vi "Test single channel GPU FFT.vi"() -> ()   [LabVIEW 2018]
panel:
  in  "stop":bool
  out "Waveform Chart":dbl(graph)
  out "error out":errorcluster
  in  "error in (no error)":errorcluster
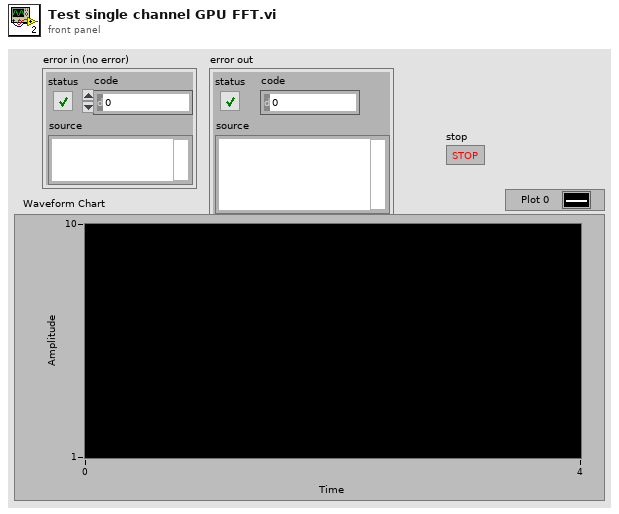
[diagram p1: front panel]
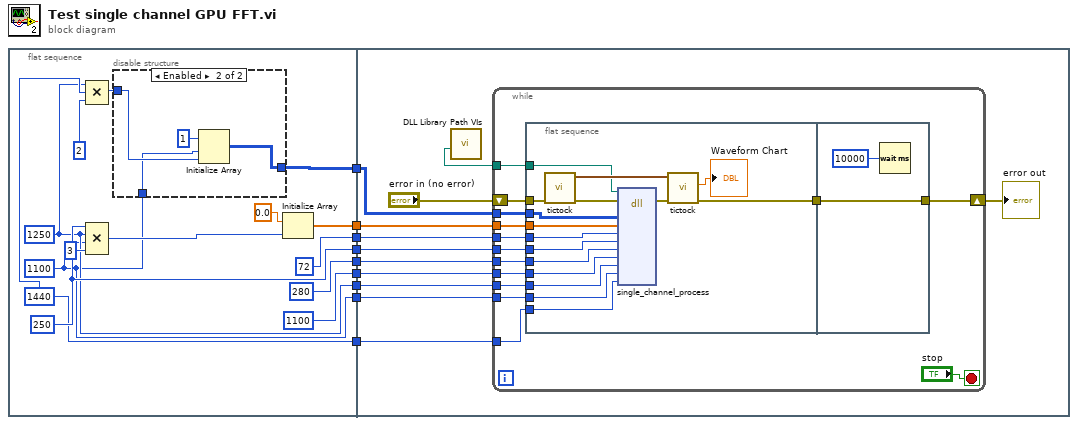
[diagram p0: block diagram]
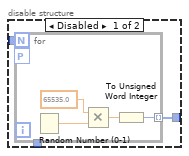
[diagram p2: hidden frame]
diagram:
  n1 = flat-sequence {
    tunnel: [w20] -> w9
    tunnel: [w19] -> w8
    tunnel: [i16 1100 ("b")] -> w7
    tunnel: [i16 280 ("a")] -> w6
    tunnel: [i16 72 ("Z0")] -> w5
    tunnel: [w15] -> w4
    tunnel: [w11] -> w3
    tunnel: [w10] -> w2
    tunnel: [w12] -> w1
    tunnel: w9 -> [w44]
    tunnel: w8 -> [w43]
    tunnel: w7 -> [w42]
    tunnel: w6 -> [w41]
    tunnel: w5 -> [w40]
    tunnel: w4 -> [w39]
    tunnel: w3 -> [w38]
    tunnel: w2 -> [w37]
    tunnel: w1 -> [w36]
    frame #0 {
      w12 = i64 1440 ("SAMPLES")
      w10 = i64 1100 ("NBLINES")
      w11 = i64 1250 ("NALINES")
      w15 = i64 250 ("DEPTH")
      n2 = Compound Arithmetic op=MULTIPLY(w11, w12, i64 2 ("value")) -> (w22:i64)
      n3 = Compound Arithmetic op=MULTIPLY(w15, w11, w10, i64 3 ("value")) -> (w23:i64)
      n4 = disable-structure shown="Enabled" {
        disable-tunnel: w22 -> [w25 w31]
        disable-tunnel: [w24 w32] -> w20
        disable-tunnel: w10 -> [_ w30]
        frame Disabled {
          n5 = for {
            N: w25 -> [_]
            tunnel: [w26] -> w24 mode=indexing
            workers-P: _ -> [_]
            n6 = Random Number (0-1)() -> (number: 0 to 1=w29:dbl)
            n7 = Multiply(x=65535.0, y=w29) -> (x*y=w27:dbl)
            n8 = To Unsigned Word Integer(number=w27) -> (unsigned 16bit integer=w26:u16)
          }
        }
        frame Enabled {
          n9 = Initialize Array(u16 1 ("element"), w30, w31) -> (w32:u16[][])
        }
      }
      n10 = Initialize Array(sgl 0.0 ("element"), w23) -> (w19:sgl[])
    }
    frame #1 {
      n11 = call "DLL Library Path VIs.vi"() -> ("GPU FFT birefringence"=w34:path)  [unwired: 6 in, 5 out]
      n12 = while {
        tunnel: w44 -> [w58]
        tunnel: w43 -> [w57]
        tunnel: w42 -> [w56]
        tunnel: w41 -> [w55]
        tunnel: w40 -> [w54]
        tunnel: w39 -> [w53]
        tunnel: w38 -> [w52]
        tunnel: w37 -> [w51]
        tunnel: w36 -> [w50]
        shift-right: [w49] -> w35
        shift-left: "error in (no error)" -> [w59]
        tunnel: w34 -> [w46]
        stop <- "stop" stop-if-true
        n13 = flat-sequence {
          tunnel: w59 -> [w75]
          tunnel: w58 -> [w60]
          tunnel: w57 -> [w74]
          tunnel: w56 -> [w73]
          tunnel: w55 -> [w72]
          tunnel: w54 -> [w71]
          tunnel: w53 -> [w70]
          tunnel: w52 -> [w69]
          tunnel: w51 -> [w68]
          tunnel: w50 -> [w67]
          tunnel: [w66] -> w47
          tunnel: w46 -> [w61]
          tunnel: [w77] -> w49
          tunnel: w47 -> [w77]
          frame #0 {
            n14 = call "tictock.vi"("error in (no error)"=w75) -> ("error out"=w65:errorcluster, "seconds since 1Jan1904"=w63:timestamp)  [unwired: 8 in, 1 out]
            n15 = dll-call lib="C:/Project/SerialSectOCT - FFT GPU/SerialSectOCT/Labview Software/DLL/CUDA_FFT_2_channel.dll" fn="single_channel_process"(path in=w61, error in=w65, "h_signal"=w60, "h_processed_signal"=w74, "Z0"=w71, "DEPTH"=w70, "a"=w72, "b"=w73, "NALINES"=w69, "NBLINES"=w68, "SAMPLES"=w67) -> (error out=w64:errorcluster)  [unwired: 11 in, 1 out]
            n16 = call "tictock.vi"("error in (no error)"=w64, "seconds since 1Jan1904 2"=w63) -> ("error out"=w66:errorcluster, "Numeric"=→"Waveform Chart":dbl)  [unwired: 7 in, 1 out]
          }
          frame #1 {
            n17 = Wait (ms)(milliseconds to wait=u32 10000) -> ()  [unwired: 1 out]
          }
        }
      }
      "error out" <- w35
    }
  }
